vi "add_Headers.vi"(8 "error in":errorcluster, 10 "headers_Add":T1, 11 "Headers In":T1) -> (0 "error out":errorcluster, 3 "Headers Out":T1)   [LabVIEW 2016]
uses:
  Headers.ctl
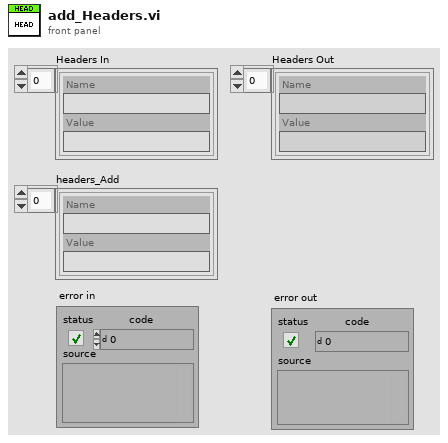
[diagram p1: front panel]
types:
  T1 = typedef "Headers.ctl" = cluster{"Name":string, "Value":string}[]
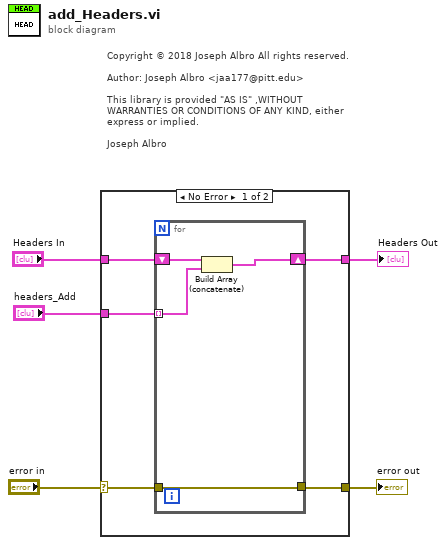
[diagram p0: block diagram]
diagram:
  # "Copyright © 2018 Joseph Albro All rights reserved.\n\nAuthor: Joseph Albro <jaa177@pitt.edu>\n\nThis library is provided \"AS IS\" ,WITHOUT WARRANTIES OR CONDITIONS OF ANY KIND, either express or implied.\n\nJoseph Albro"
  n1 = case shown="No Error" "error in" {
    selector: "error in" -> [w9 w14]
    tunnel: [w9 w14] -> w5
    tunnel: "Headers In" -> [w8 w15]
    tunnel: "headers_Add" -> [w7 _]
    tunnel: [w6 w15] -> w1
    frame No Error {
      n2 = for {
        tunnel: w9 -> [w13]
        tunnel: [w13] -> _
        shift-right: [w11] -> w6
        shift-left: w8 -> [w12]
        tunnel: w7 -> [w10] mode=indexing
        n3 = Build Array (concatenate)(w12, w10) -> (w11:T1)
      }
    }
    frame Error {
    }
  }
  "error out" <- w5
  "Headers Out" <- w1
